vi "8-Tap 8-bit Camera with Serial Server with Debugging(FPGA).vi"() -> ()   [LabVIEW 2013]
doc: "This is the FPGA VI for the 10-Tap 8-Bit Camera with DRAM example. This example demonstrates how to acquire images from a 10-tap, 8-bit, extended configuration, Camera Link camera and transfer the images to the host. This example supports area scan and line scan cameras for both continuous and finite acquisitions.\n\nThis example also demonstrates the use of DRAM as a frame buffer for very high speed acquisitions. Data packing and flow-control are also employed to maximize use of the available DRAM and FIFOs in terms of both memory space and performance.\n\nAdditionally, the example demonstrates the serial server, which allows third-party camera configuration utilities to communicate with the camera using the Camera Link serial interface while this VI is running."
uses:
  Common/CL Signal Mapping.ctl
  Common/CL Configuration.ctl
  FPGA/Sector/Accumulate/Sector Parameter Cluster.ctl
  <vilib>/Platform/TimedLoop/XDataNode/timing_clust.ctl
  <vilib>/Platform/TimedLoop/XDataNode/nitl_modes.ctl
  <vilib>/Platform/TimedLoop/XDataNode/wakeup.ctl
  <vilib>/rvi/Emulation/niFpgaSctlEmulationGetInTimedLoop.vi
  <vilib>/rvi/Emulation/niFpgaEmulationReportErrorSimple.vi
  <vilib>/rvi/eio/common/nirviEmuTemplateMethod_errors.vi
  <vilib>/rvi/Emulation/niFpgaGetClockAttributes.vi
  <vilib>/rvi/Emulation/niFpgaCriticalErrorInLSC.vi
  <vilib>/rvi/FIFO/Fifo_Resource/nirvififoEmulationReadFpgaImpl.vi
  <vilib>/rvi/DataTransferAndStorage/Container/Common/niFpgaContainerGetUniqueNameForEmu.vi
  Common/CL Data to Pixels/8 Tap 8-Bit.vi
  <vilib>/rvi/FIFO/Fifo_Resource/nirvififoEmulationWriteFpgaImpl.vi
  <vilib>/rvi/interface/RandomDataEmulation/nirviRandomDataFPGAFIFO.vi
  <vilib>/rvi/interface/RandomDataEmulation/niFpgaRandomDataHandleErrors.vi
  <vilib>/rvi/FIFO/Fifo_Resource/nirvififoEmulationGetNumberOfElementsToReadFpgaImpl.vi
  <vilib>/rvi/FIFO/Fifo_Resource/nirvififoEmulationGetNumberOfElementsToWriteFpgaImpl.vi
  <vilib>/rvi/Emulation/niFpgaProcessEmulError.vi
  FPGA/Globals/Sector Parameter Global.vi
  FPGA/Globals/Pixel Location Global.vi
  FPGA/Globals/Accumulated Sector Intensity.vi
  <vilib>/Platform/TimedLoop/XDataNode/XDataNode.xnode
  <vilib>/eio/EIONode/EIONode.xnode
  <vilib>/rvi/DataTransferAndStorage/Container/XNode/niFpgaContainer.xnode
  <vilib>/rvi/FIFO/Fifo_Resource/nirvififoEmulationRead.vi
  <vilib>/rvi/FIFO/Fifo_Resource/nirvififoEmulationWrite.vi
  <vilib>/rvi/interface/RandomDataEmulation/nirviRandomDataFpgaReadWriteTemplate.vi
  <vilib>/rvi/FIFO/Fifo_Resource/nirvififoEmulationGetNumberOfElementsToRead.vi
  <vilib>/rvi/FIFO/Fifo_Resource/nirvififoEmulationGetNumberOfElementsToWrite.vi
  <vilib>/Platform/TimedLoop/XDataNode/XDNodeRunTimeDep.lvlib
panel:
  out "Data":bool
  out "Sector Group TO":bool
  out "Host DMA TO":bool
  out "Cam Data 64 TO":bool
  out "Number of Elements to Write Sector Grouping":u32
  out "Accumulated":T1(array[cluster])
  out "Analysis Ticks":u32
  out "Right Sector Edge":u8
  out "Left Sector Edge":u8
  in  "# of Frames to Average":u8
  in  "Sector Parameters Left":T2={"Start Angle"=0.65740966796875, "End Angle"=0.99468994140625, "Inner Radius"=309, "Outter Radius"=405, "Hinge X"=464, "Hinge Y"=534, "NumWingSectors"=8}
  in  "Sector Parameters Right":T2={"Start Angle"=0.0, "End Angle"=0.4708251953125, "Inner Radius"=309, "Outter Radius"=405, "Hinge X"=685, "Hinge Y"=527, "NumWingSectors"=8}
  in  "Sector Threshold":u8
  in  "[Average BG Intensity]":u8[](array[numeric])=[0, 0, 0, 0, 0, 0, 0, 0, 0, 0, 0, 0, 0, 0, 0, 0, 0, 0, 0, 0, 0, 0, 0, 0, 0, 0, 0, 0, 0, 0, 0, 0]
  in  "X Resolution":u16=1000
  in  "Y Resolution":u16=1000
  in  "Left Start Angle Duty Cycle":fxp<+,8,0>
  in  "Left End Angle Duty Cycle":fxp<+,8,0>
  in  "Right Start Angle Duty Cycle":fxp<+,8,0>
  in  "Right End Angle Duty Cycle":fxp<+,8,0>
  out "Number of Elements to Write Host DMA":u32
  out "Number of Elements to Read Cam Data":u32
  in  "CL Config.Configuration":T3=enum."Full"
  in  "CL Config.Signal Mapping":T4
  in  "CL Config.Line Scan":bool
  in  "CL Config.DVAL Active High":bool=TRUE
  in  "CL Config.LVAL Active High":bool=TRUE
  in  "CL Config.FVAL Active High":bool=TRUE
  in  "CL Config.Spare Active High":bool=TRUE
  in  "Acq Control.Line Scan Height":u32
  in  "Acq Control.Frames To Acq":u32
  in  "Acq Control.Acquire":bool
  in  "Acq Control.Cancel Acq":bool
  in  "Acq Control.Ignore DVAL":bool
  in  "Acq Control.Initialize":bool
  out "Acq Status.Acq In Progress":bool
  out "Acq Status.Clocks Per Line":u32
  out "Acq Status.Frames Acq'd":u32
  out "Acq Status.Lines Per Frame":u32
  out "Acq Status.DMA Write Timeout":bool
  out "Acq Status.Initialized":bool
  in  "UART.Baud Rate":u8
  in  "UART.Transmit":bool
  in  "UART.Tx Data":u8[](array[numeric])=[0, 0, 0, 0, 0, 0, 0, 0, 0, 0] format="%02x"
  in  "UART.Set Baud Rate":bool
  in  "UART.Byte Mode":bool=TRUE
  out "UART.Rx Ready":bool
  out "UART.Break Indicator":bool
  out "UART.Framing Error":bool
  out "UART.Overrun Error":bool
  out "UART.Tx Ready":bool
  out "UART.Rx Data":u8 format="%02x"
  in  "UART.Receive":bool
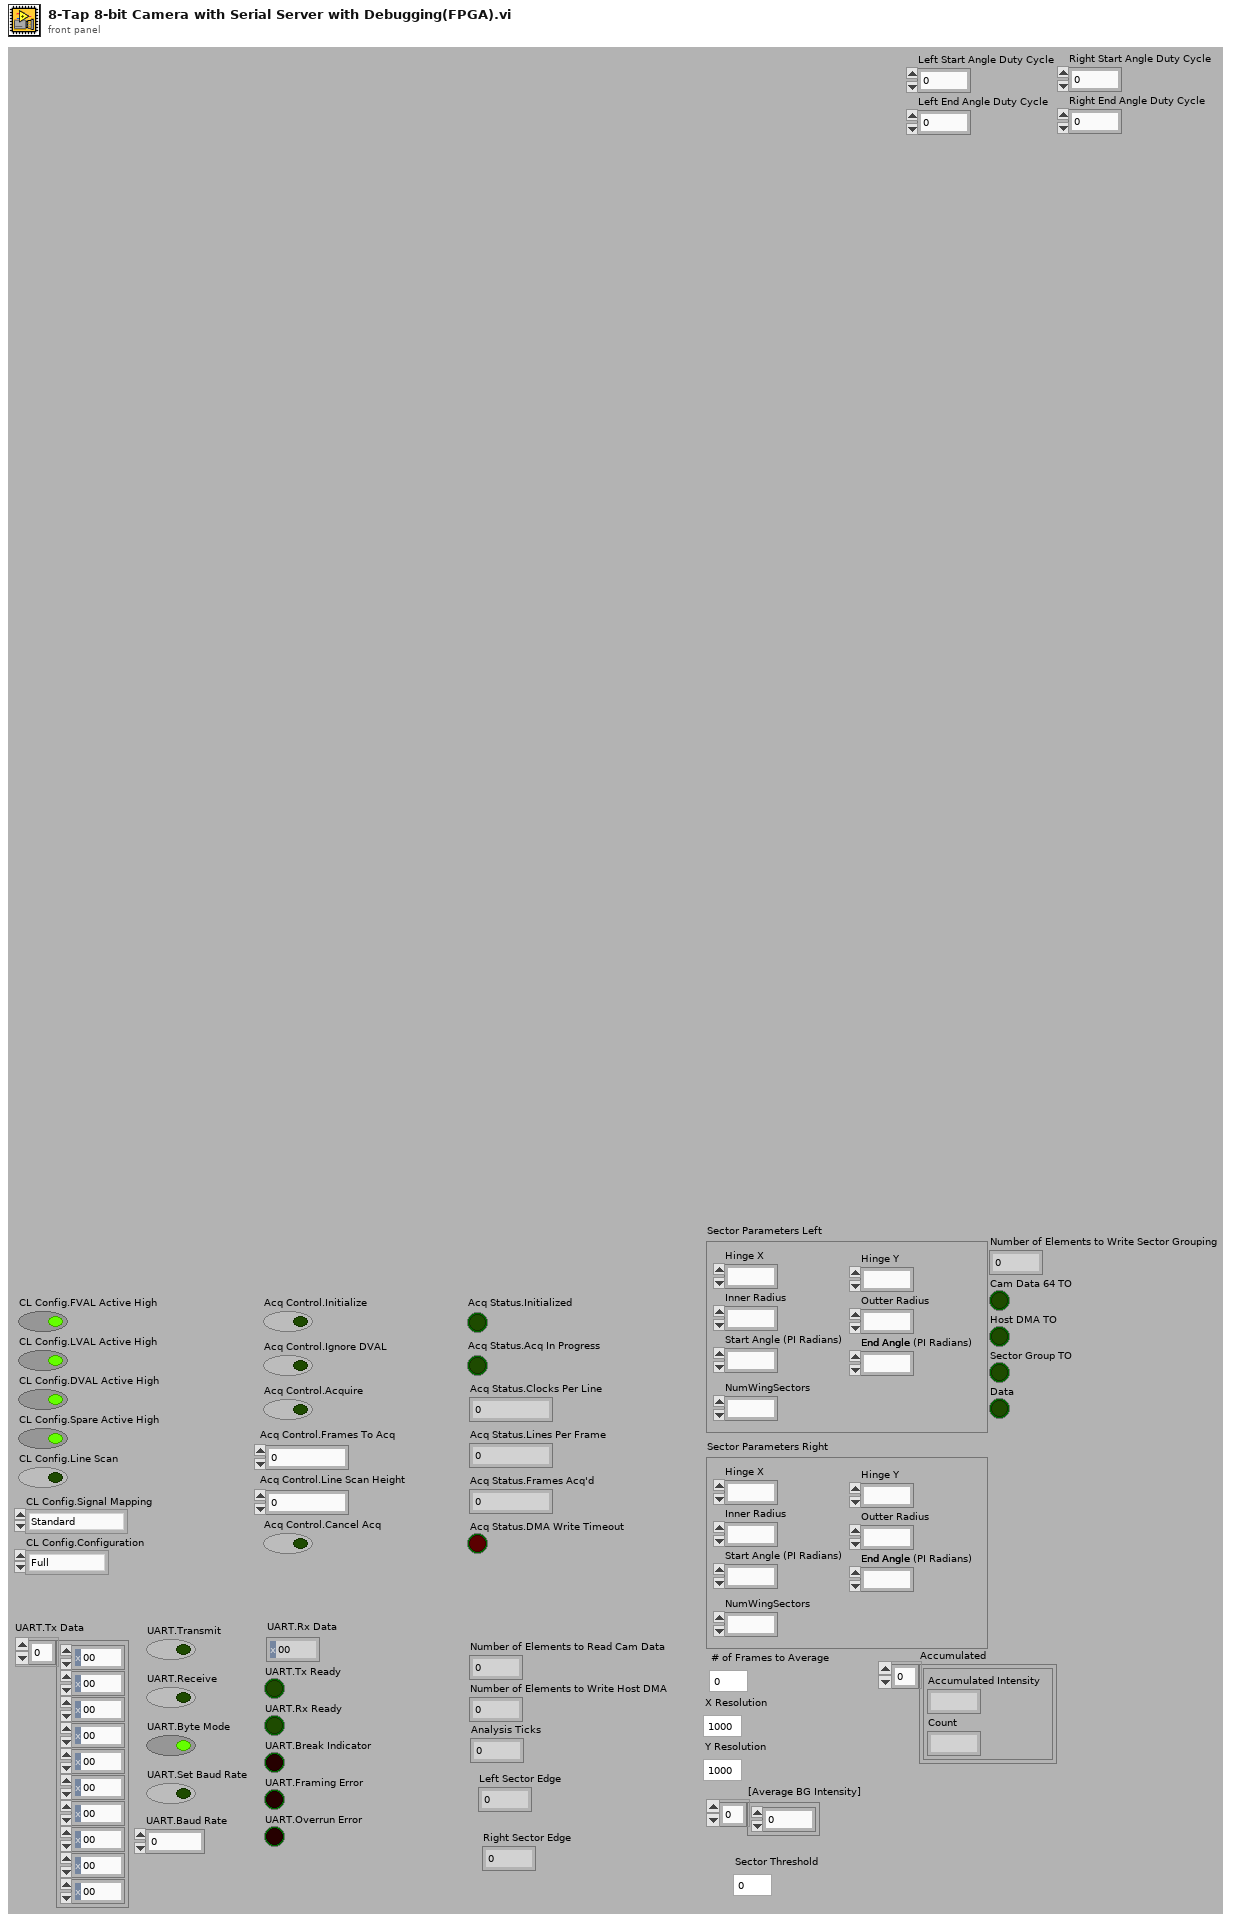
[diagram p1: front panel]
types:
  T1 = cluster{"Accumulated Intensity":fxp<+,20,20>, "Count":fxp<+,12,12>}[]
  T2 = typedef "Sector Parameter Cluster.ctl" = cluster{"Start Angle":fxp<+/-,17,2>, "End Angle":fxp<+,17,3>, "Inner Radius":u16, "Outter Radius":u16, "Hinge X":u16, "Hinge Y":u16, "NumWingSectors":u8}
  T3 = typedef "CL Configuration.ctl" = enum8{"Base", "Medium", "Full"}
  T4 = typedef "CL Signal Mapping.ctl" = enum8{"Standard", "Basler 10-tap", "Vosskühler 10-tap"}
  T5 = typedef "XDNodeRunTimeDep.lvlib/timing_clust.ctl" = cluster{"Expected End [f-1]":u64, "Actual End [f-1]":u64, "Finished Late? [f-1]":bool, "Expected End [i-1]":u64, "Actual End [i-1]":u64, "Finished Late? [i-1]":bool, "Expected Start [i]":u64, "Actual Start [i]":u64, "Expected Start [f]":u64, "Actual Start [f]":u64, "Source Name":string, "Structure Name":string, "Period":i64, "Deadline":i64, "Offset":i64, "Start":i64, "Priority":i32, "Timeout":i32, "Mode":T6, "Wakeup Reason":T7, "Error":errorcluster, "Source Type":string, "Secondary Source Type":string, "Global End Time":u64, "Global Start Time":u64, "Frame Duration":u64, "Iteration Duration":u64, "Assigned CPU":i32, "I/O Scan Engine Mode":u32}
  T6 = typedef "XDNodeRunTimeDep.lvlib/nitl_modes.ctl" = enum32{"No Change", "Process missed periods, maintain original phase", "Discard missed periods, maintain original phase", "Process missed periods, ignore original phase", "Discard missed periods, ignore original phase"}
  T7 = typedef "XDNodeRunTimeDep.lvlib/wakeup.ctl" = enum32{"Normal", "Aborted", "Asynchronous wakeup", "Timing source error", "Timed loop error", "Timeout"}
  T8 = cluster{"Enables Valid":bool, "Frame Valid":bool, "Line Valid":bool, "Data Valid":bool}
  T9 = cluster{"Pixel 0":u8, "Pixel 1":u8, "Pixel 2":u8, "Pixel 3":u8, "Pixel 4":u8, "Pixel 5":u8, "Pixel 6":u8, "Pixel 7":u8}
  T10 = cluster{"Tx Data":u8[], "Transmit":bool, "Receive":bool, "Byte Mode":bool, "Set Baud Rate":bool, "Baud Rate":u8}
  T11 = cluster{"Rx Data":u8, "Turn Off Transmit":bool, "Turn Off Receive":bool, "Turn Off Set Baud Rate":bool, "Tx Ready":bool, "Rx Ready":bool, "Break Indicator":bool, "Framing Error":bool, "Overrun Error":bool}
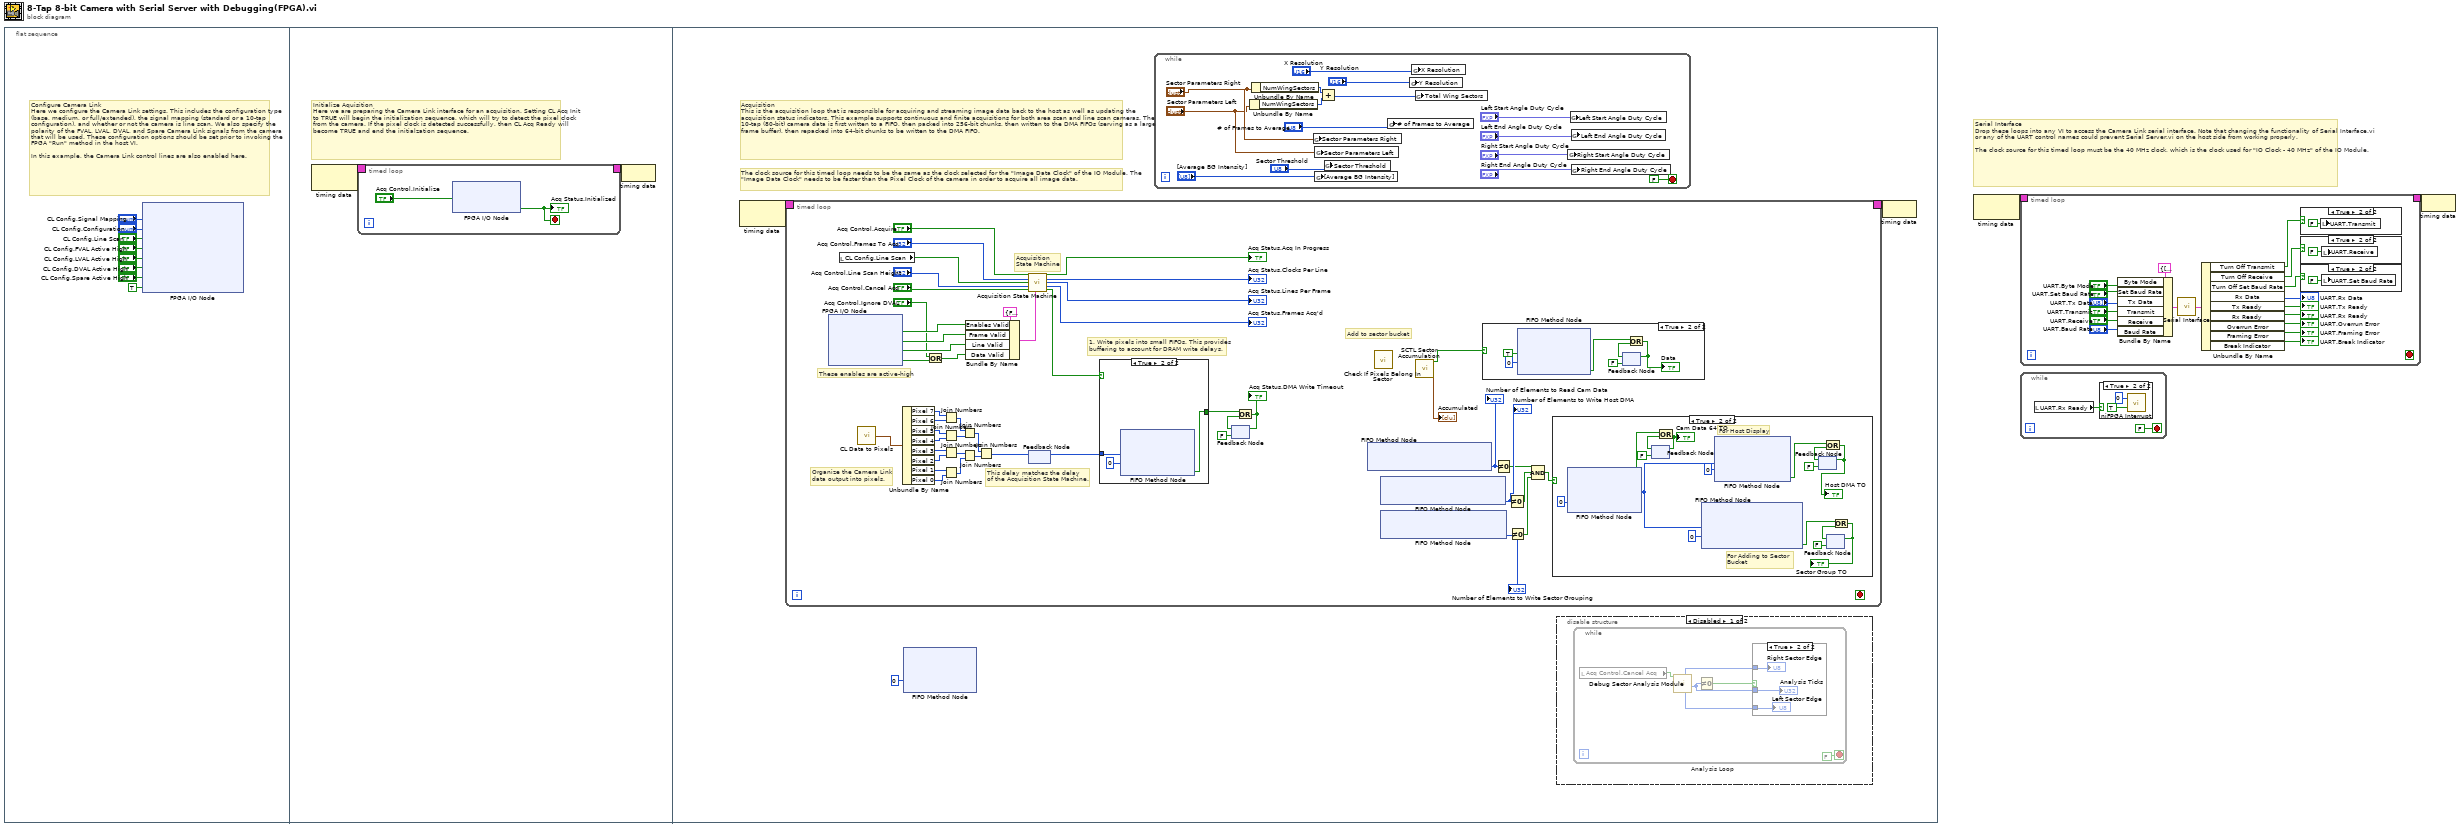
[diagram p0: block diagram]
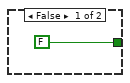
[diagram p10: hidden frame]
diagram:
  # "Serial Interface\nDrop these loops into any VI to access the Camera Link serial interface. Note that changing the functionality of Serial Interface.vi or any of the UART control names could prevent Serial Server.vi on the host side from working properly.\n\nThe clock source for this timed loop must be the 40 MHz clock, which is the clock used for \"IO Clock - 40 MHz\" of the IO Module."
  n1 = flat-sequence {
    frame #0 {
      # "Configure Camera Link\nHere we configure the Camera Link settings. This includes the configuration type (base, medium, or full/extended), the signal mapping (standard or a 10-tap configuration), and whether or not the camera is line scan. We also specify the polarity of the FVAL, LVAL, DVAL, and Spare Camera Link signals from the camera that will be used. These configuration options should be set prior to invoking the FPGA \"Run\" method in the host VI.\n\nIn this example, the Camera Link control lines are also enabled here."
      n2 = xnode "FPGA I/O Node"("CL Set Signal Mapping"="CL Config.Signal Mapping", "CL Set Configuration"="CL Config.Configuration", "CL Set Line Scan"="CL Config.Line Scan", "CL Set FVAL Active High"="CL Config.FVAL Active High", "CL Set LVAL Active High"="CL Config.LVAL Active High", "CL Set DVAL Active High"="CL Config.DVAL Active High", "CL Set Spare Active High"="CL Config.Spare Active High", "CL Control Enable"=TRUE ("IO Module\\CL Control Enable")) -> ()  [unwired: 8 in, 8 out]
    }
    frame #1 {
      # "Initialize Aquisition\nHere we are preparing the Camera Link interface for an acquisition. Setting CL Acq Init to TRUE will begin the initialization sequence, which will try to detect the pixel clock from the camera. If the pixel clock is detected successfully, then CL Acq Ready will become TRUE and end the initialzation sequence."
      n3 = node-c288() -> (w12:T5)  [unwired: 1 out]
      n4 = timed-loop {
        timing: w12 -> [_]
        timing-out: [_] -> w11
        stop <- w13 stop-if-true
        n5 = xnode "FPGA I/O Node"("CL Acq Init"="Acq Control.Initialize") -> ("CL Acq Ready"=w13:bool)  [unwired: 2 in, 2 out]
        "Acq Status.Initialized" <- w13
      }
      n6 = node-c288(w11) -> ()
    }
    frame #2 {
      # "The clock source for this timed loop needs to be the same as the clock selected for the \"Image Data Clock\" of the IO Module. The \"Image Data Clock\" needs to be faster than the Pixel Clock of the camera in order to acquire all image data."
      # "Acquisition\nThis is the acquisition loop that is responsible for acquiring and streaming image data back to the host as well as updating the acquisition status indicators. This example supports continuous and finite acquisitions for both area scan and line scan cameras. The 10-tap (80-bit) camera data is first written to a FIFO, then packed into 256-bit chunks, then written to the DMA FIFOs (serving as a large frame buffer), then repacked into 64-bit chunks to be written to the DMA FIFO."
      n7 = node-c288() -> (w21:T5)  [unwired: 1 in]
      n8 = timed-loop {
        timing: w21 -> [_]
        timing-out: [_] -> w20
        stop <- _ stop-if-true
        # "Add to sector bucket"
        # "1. Write pixels into small FIFOs. This provides\nbuffering to account for DRAM write delays."
        # "Organize the Camera Link\ndata output into pixels."
        # "These enables are active-high"
        # "This delay matches the delay\nof the Acquisition State Machine."
        # "Acquisition\nState Machine"
        n9 = xnode "FPGA I/O Node"() -> ("CL Output Valid"=w79:bool, "CL Frame Valid"=w78:bool, "CL Line Valid"=w77:bool, "CL Data Valid"=w74:bool)  [unwired: 4 in, 4 out]
        n10 = local read "CL Config.Line Scan"() -> (w71:bool)
        n11 = call-poly "CL Data to Pixels.vi"() -> ("Pixels"=w93:T9)  [unwired: 1 in]
        n12 = Unbundle By Name(w93) -> ("Pixel 7"=w69:u8, "Pixel 6"=w68:u8, "Pixel 5"=w67:u8, "Pixel 4"=w66:u8, "Pixel 3"=w65:u8, "Pixel 2"=w64:u8, "Pixel 1"=w63:u8, "Pixel 0"=w62:u8)
        n13 = Or(x="Acq Control.Ignore DVAL", y=w74) -> (x .or. y?=w73:bool)
        n14 = Join Numbers(hi=w69, lo=w68) -> ((hi.lo)=w60:u16)
        n15 = Join Numbers(hi=w67, lo=w66) -> ((hi.lo)=w59:u16)
        n16 = Join Numbers(hi=w65, lo=w64) -> ((hi.lo)=w58:u16)
        n17 = Join Numbers(hi=w63, lo=w62) -> ((hi.lo)=w61:u16)
        n18 = Join Numbers(hi=w60, lo=w59) -> ((hi.lo)=w57:u32)
        n19 = Join Numbers(hi=w58, lo=w61) -> ((hi.lo)=w56:u32)
        n20 = Bundle By Name(cluster=T8 {"Enables Valid"=FALSE, "Frame Valid"=FALSE, "Line Valid"=FALSE, "Data Valid"=FALSE} ("Enables"), "Enables Valid"=w79, "Frame Valid"=w78, "Line Valid"=w77, "Data Valid"=w73) -> (w76:T8)
        n21 = Join Numbers(hi=w57, lo=w56) -> ((hi.lo)=w55:u64)
        n22 = call "Acquisition State Machine.vi"("Acquire"="Acq Control.Acquire", "Frames to Acquire"="Acq Control.Frames To Acq", "Line Scan"=w71, "Line Scan Height"="Acq Control.Line Scan Height", "Cancel Acq"="Acq Control.Cancel Acq", "Enables"=w76) -> ("Acq In Progress"=→"Acq Status.Acq In Progress":bool, "Num Clocks Per Line"=→"Acq Status.Clocks Per Line":u32, "Num Lines Per Frame"=→"Acq Status.Lines Per Frame":u32, "Num Frames Acq'd"=→"Acq Status.Frames Acq'd":u32, "Capture Cycle"=w91:bool)  [unwired: 4 in, 1 out]
        n23 = feedback-in #1(w55) -> ()
        n24 = feedback #1() -> (w92:u64)  [unwired: 1 in]
        n25 = case shown="True" w91 {
          tunnel: [FALSE ("Timed Out?") w118] -> w89
          tunnel: w92 -> [_ w119]
          frame False {
          }
          frame True {
            n26 = xnode ("FIFO Method Node")("Element"=w119, "Timeout"=0) -> ("Timed Out?"=w118:bool)  [unwired: 1 in, 1 out]
          }
        }
        n27 = feedback #2(FALSE) -> (w88:bool)
        n28 = Or(x=w89, y=w88) -> (x .or. y?=w87:bool)
        "Acq Status.DMA Write Timeout" <- w87
        n29 = feedback-in #2(w87) -> ()
        n30 = xnode ("FIFO Method Node")() -> ("Number of Elements to Read"=w53:u32)  [unwired: 1 in, 1 out]
        "Number of Elements to Read Cam Data" <- w53
        n31 = call "Check If Pixels Belong In Sector.vi"() -> ()  [unwired: 11 in, 1 out]
        n32 = xnode ("FIFO Method Node")() -> ("Number of Elements to Write"=w51:u32)  [unwired: 1 in, 1 out]
        "Number of Elements to Write Host DMA" <- w51
        n33 = xnode ("FIFO Method Node")() -> ("Number of Elements to Write"=w50:u32)  [unwired: 1 in, 1 out]
        "Number of Elements to Write Sector Grouping" <- w50
        n34 = call "SCTL Sector Accumulation.vi"() -> ("Accummulated"=→"Accumulated":T1, "New Data?"=w54:bool)  [unwired: 10 in]
        n35 = case shown="True" w54 {
          frame False {
          }
          frame True {
            n36 = xnode ("FIFO Method Node")("Element"=TRUE, "Timeout"=0) -> ("Timed Out?"=w111:bool)  [unwired: 1 in, 1 out]
            n37 = feedback #3(FALSE) -> (w112:bool)
            n38 = Or(x=w111, y=w112) -> (x .or. y?=w110:bool)
            "Data" <- w110
            n39 = feedback-in #3(w110) -> ()
          }
        }
        n40 = Not Equal To 0?(x=w53) -> (x != 0?=w48:bool)
        n41 = Not Equal To 0?(x=w51) -> (x != 0?=w52:bool)
        n42 = Not Equal To 0?(x=w50) -> (x != 0?=w49:bool)
        n43 = Compound Arithmetic op=AND(w48, w52, w49) -> (w47:bool)
        n44 = case shown="True" w47 {
          frame False {
          }
          frame True {
            # "For Adding to Sector \nBucket"
            # "For Host Display"
            n45 = xnode ("FIFO Method Node")("Timeout"=0) -> ("Element"=w106:u64, "Timed Out?"=w95:bool)  [unwired: 1 in, 1 out]
            n46 = feedback #4(FALSE) -> (w97:bool)
            n47 = Or(x=w95, y=w97) -> (x .or. y?=w94:bool)
            "Cam Data 64 TO" <- w94
            n48 = feedback-in #4(w94) -> ()
            n49 = xnode ("FIFO Method Node")("Element"=w106, "Timeout"=0) -> ("Timed Out?"=w99:bool)  [unwired: 1 in, 1 out]
            n50 = xnode ("FIFO Method Node")("Element"=w106, "Timeout"=0) -> ("Timed Out?"=w103:bool)  [unwired: 1 in, 1 out]
            n51 = feedback #5(FALSE) -> (w104:bool)
            n52 = Or(x=w103, y=w104) -> (x .or. y?=w102:bool)
            "Host DMA TO" <- w102
            n53 = feedback-in #5(w102) -> ()
            n54 = feedback #6(FALSE) -> (w100:bool)
            n55 = Or(x=w99, y=w100) -> (x .or. y?=w98:bool)
            "Sector Group TO" <- w98
            n56 = feedback-in #6(w98) -> ()
          }
        }
      }
      n57 = xnode ("FIFO Method Node")("Timeout"=0) -> ()  [unwired: 1 in, 3 out]
      n58 = while {
        stop <- FALSE stop-if-true
        n59 = Unbundle By Name("Sector Parameters Left") -> ("NumWingSectors"=w43:u8)
        n60 = Unbundle By Name("Sector Parameters Right") -> ("NumWingSectors"=w44:u8)
        n61 = global write "Sector Parameter Global.vi" "Sector Parameters Right"("Sector Parameters Right") -> ()
        n62 = global write "Sector Parameter Global.vi" "Sector Parameters Left"("Sector Parameters Left") -> ()
        n63 = global write "Sector Parameter Global.vi" "[Average BG Intensity]"("[Average BG Intensity]") -> ()
        n64 = Add(x=w44, y=w43) -> (x+y=w42:u8)
        n65 = global write "Sector Parameter Global.vi" "Sector Threshold"("Sector Threshold") -> ()
        n66 = global write "Pixel Location Global.vi" "# of Frames to Average"("# of Frames to Average") -> ()
        n67 = global write "Pixel Location Global.vi" "Y Resolution"("Y Resolution") -> ()
        n68 = global write "Pixel Location Global.vi" "X Resolution"("X Resolution") -> ()
        n69 = global write "Accumulated Sector Intensity.vi" "Total Wing Sectors"(w42) -> ()
        n70 = global write "Sector Parameter Global.vi" "Right Start Angle Duty Cycle"("Right Start Angle Duty Cycle") -> ()
        n71 = global write "Sector Parameter Global.vi" "Left Start Angle Duty Cycle"("Left Start Angle Duty Cycle") -> ()
        n72 = global write "Sector Parameter Global.vi" "Left End Angle Duty Cycle"("Left End Angle Duty Cycle") -> ()
        n73 = global write "Sector Parameter Global.vi" "Right End Angle Duty Cycle"("Right End Angle Duty Cycle") -> ()
      }
      n74 = disable-structure shown="Disabled" {
        frame Disabled {
          n75 = while "Analysis Loop" {
            stop <- FALSE stop-if-true
            n76 = local read "Acq Control.Cancel Acq"() -> (w26:bool)
            n77 = call "Debug Sector Analysis Module.vi"("Canceled?"=w26) -> ("Analysis Ticks"=w25:u32, "Left Sector Edge"=w22:u8, "Right Sector Edge"=w23:u8)  [unwired: 6 in, 2 out]
            n78 = Not Equal To 0?(x=w25) -> (x != 0?=w24:bool)
            n79 = case shown="True" w24 {
              tunnel: w25 -> [_ w30]
              tunnel: w23 -> [_ w29]
              tunnel: w22 -> [_ w28]
              frame False {
              }
              frame True {
                "Analysis Ticks" <- w30
                "Right Sector Edge" <- w29
                "Left Sector Edge" <- w28
              }
            }
          }
        }
        frame Enabled {
        }
      }
      n80 = node-c288(w20) -> ()
    }
  }
  n81 = node-c288() -> (w2:T5)  [unwired: 1 out]
  n82 = timed-loop {
    timing: w2 -> [_]
    timing-out: [_] -> w1
    stop <- _ stop-if-true
    n83 = Bundle By Name(cluster=T10 {"Tx Data"=[0, 0, 0, 0, 0, 0, 0, 0, 0, 0], "Transmit"=FALSE, "Receive"=FALSE, "Byte Mode"=TRUE, "Set Baud Rate"=FALSE, "Baud Rate"=0} ("UART Inputs"), "Byte Mode"="UART.Byte Mode", "Set Baud Rate"="UART.Set Baud Rate", "Tx Data"="UART.Tx Data", "Transmit"="UART.Transmit", "Receive"="UART.Receive", "Baud Rate"="UART.Baud Rate") -> (w124:T10)
    n84 = call "Serial Interface.vi"("UART Inputs"=w124) -> ("UART Outputs"=w136:T11)
    n85 = Unbundle By Name(w136) -> ("Turn Off Transmit"=w129:bool, "Turn Off Receive"=w130:bool, "Turn Off Set Baud Rate"=w126:bool, "Rx Data"=→"UART.Rx Data":u8, "Tx Ready"=→"UART.Tx Ready":bool, "Rx Ready"=→"UART.Rx Ready":bool, "Overrun Error"=→"UART.Overrun Error":bool, "Framing Error"=→"UART.Framing Error":bool, "Break Indicator"=→"UART.Break Indicator":bool)
    n86 = case shown="True" w129 {
      frame False {
      }
      frame True {
        n87 = local write "UART.Transmit"(FALSE ("UART.Transmit")) -> ()
      }
    }
    n88 = case shown="True" w130 {
      frame False {
      }
      frame True {
        n89 = local write "UART.Receive"(FALSE ("UART.Receive")) -> ()
      }
    }
    n90 = case shown="True" w126 {
      frame False {
      }
      frame True {
        n91 = local write "UART.Set Baud Rate"(FALSE ("UART.Receive")) -> ()
      }
    }
  }
  n92 = while {
    stop <- FALSE stop-if-true
    n93 = local read "UART.Rx Ready"() -> (w148:bool)
    n94 = case shown="True" w148 {
      frame False {
      }
      frame True {
        n95 = call <vilib>:"niFPGA Interrupt.vi"("Wait Until Cleared (F)"=TRUE ("Wait Until Cleared"), "IRQ Number (0)"=u8 0 ("IRQ Number")) -> ()  [unwired: 1 in]
      }
    }
  }
  n96 = node-c288(w1) -> ()
